vi "ContinousLoopMain.vi"(0 "ProgramPathInput":path, 11 "error in":errorcluster) -> (2 "Output Directory":path, 3 "File Prefix":string, 4 "Total Duration":dbl format="%<%H:%M:%S>t", 6 "Interval":dbl format="%<%H:%M:%S>t", 10 "Microscope":T1(array[cluster]), 12 "ProgramStopped":bool, 13 "StartProgram":bool, 14 "Positions":dbl[][](array[numeric]), 15 "error out":errorcluster)   [LabVIEW 2018, in "ContinousLoop.lvlib"]
uses:
  ContinousLoop.lvlib
  Config/Config.lvlib
panel:
  in  "Start Program":bool
  in  "stop":bool
  in  "Configuration File":path
  out "Continuous Program":string[][](array[string])
  # "Microscope"
  # "Program Control"
  # "Positions"
  # "Steps"
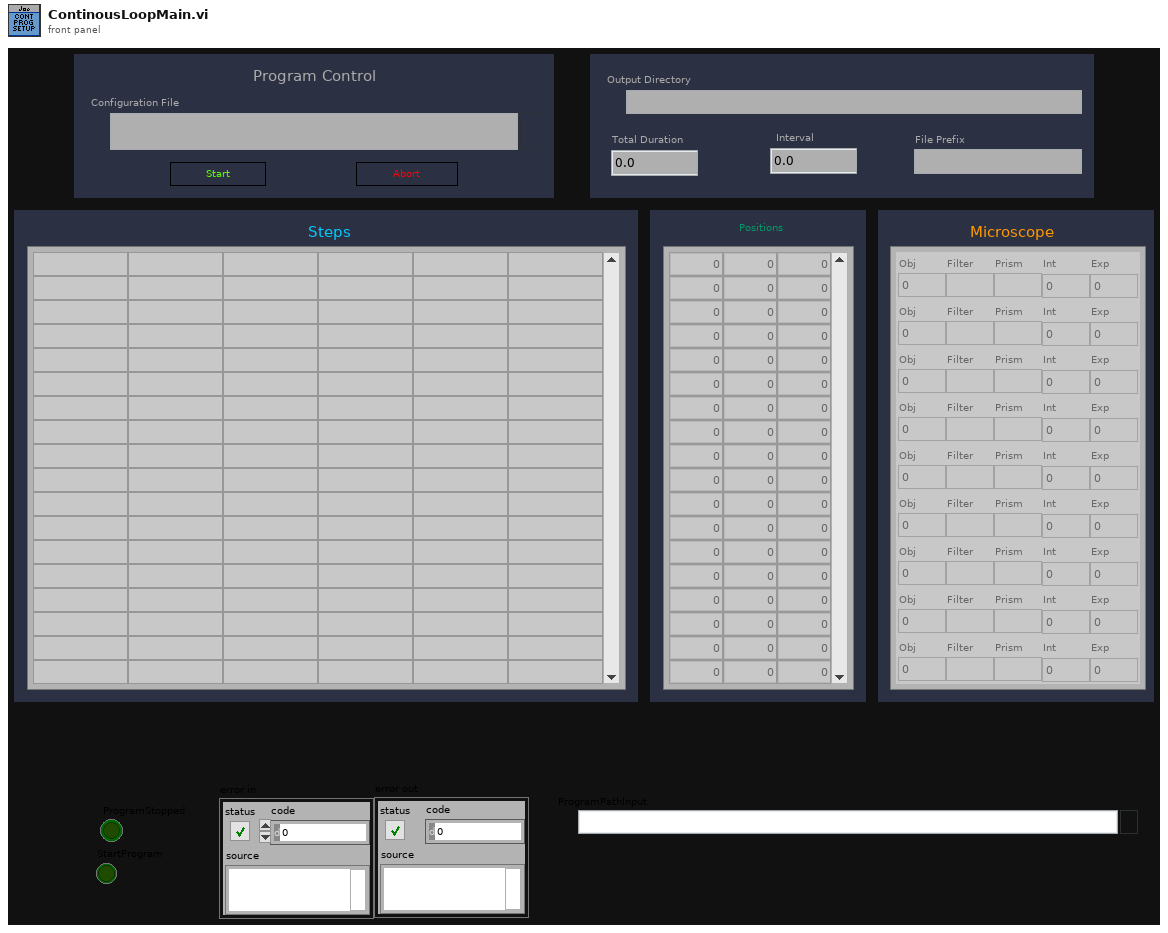
[diagram p1: front panel]
types:
  T1 = cluster{"Obj":i32, "Filter":string, "Prism":string, "Int":dbl, "Exp":i32}[]
  T2 = cluster{"Objective":i32, "Filter":string, "Prism":string, "Intensity":dbl, "Exposure":i32}[]
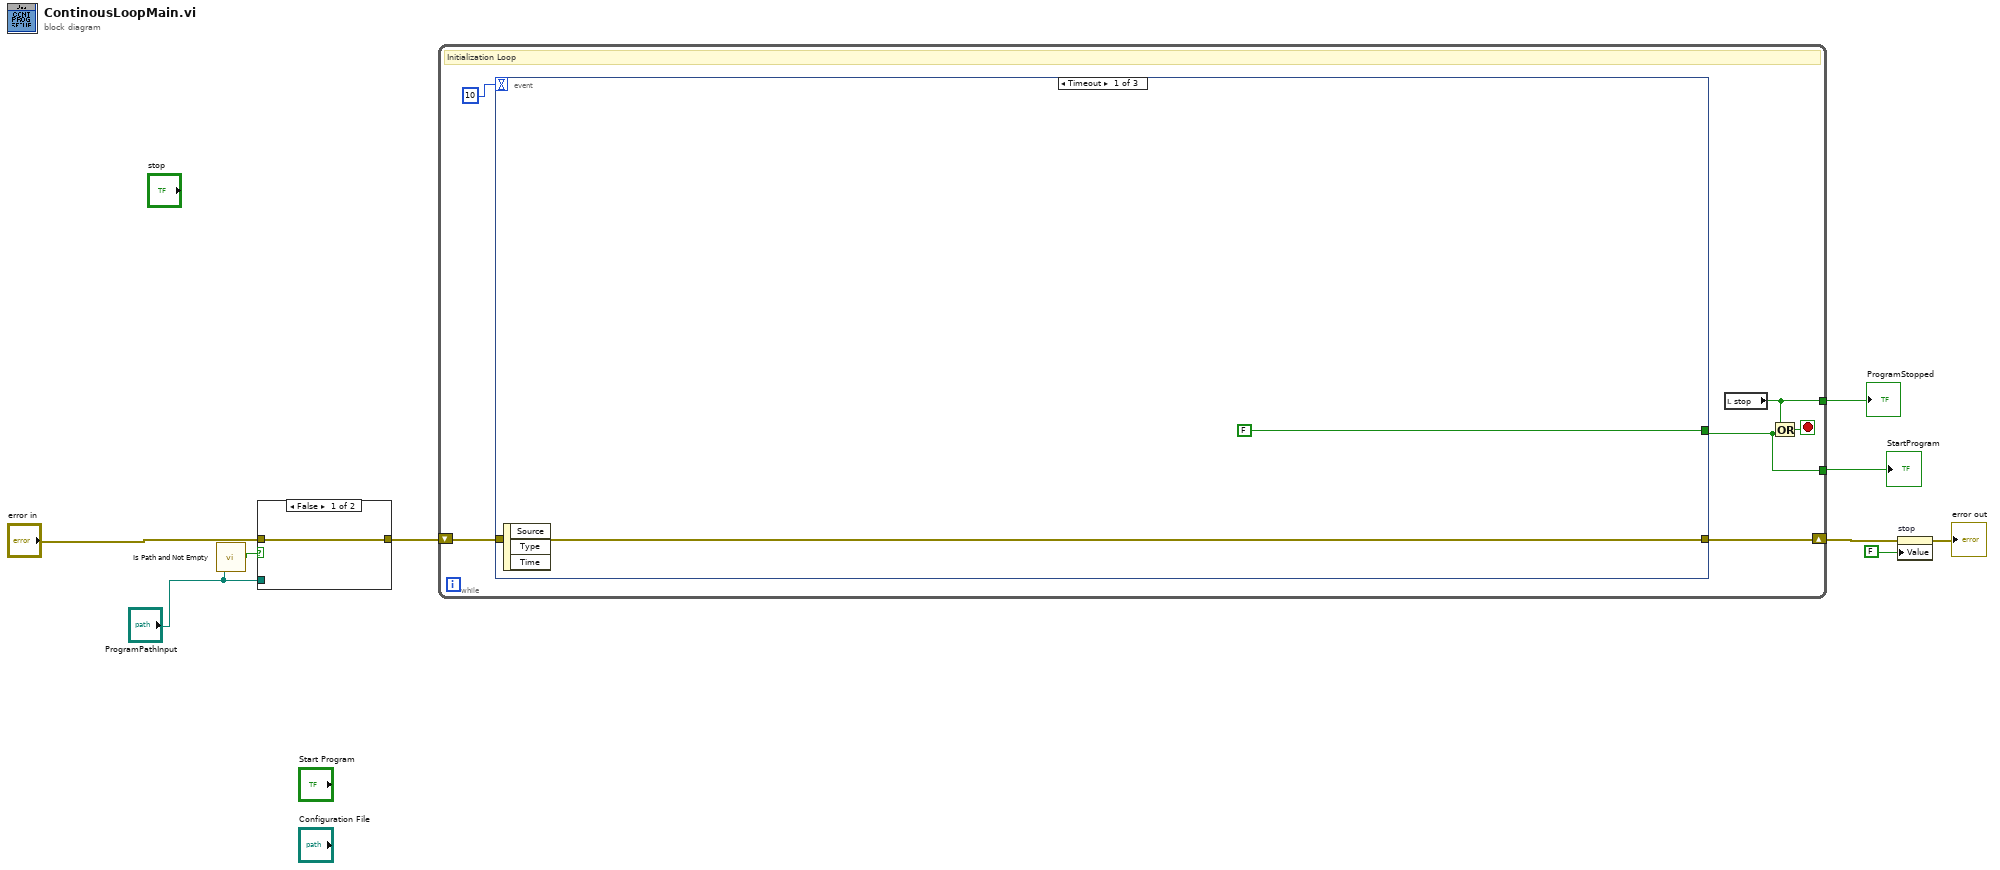
[diagram p0: block diagram]
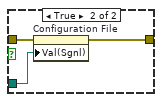
[diagram p2: hidden frame]
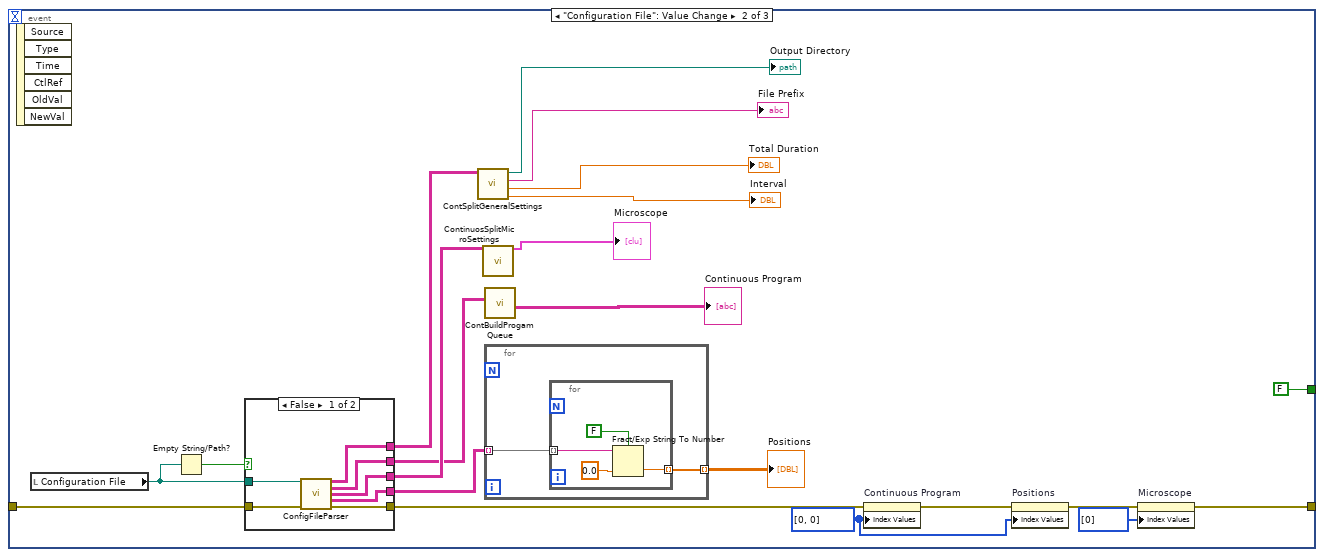
[diagram p3: hidden frame]
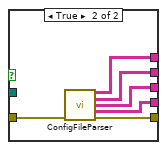
[diagram p4: hidden frame]
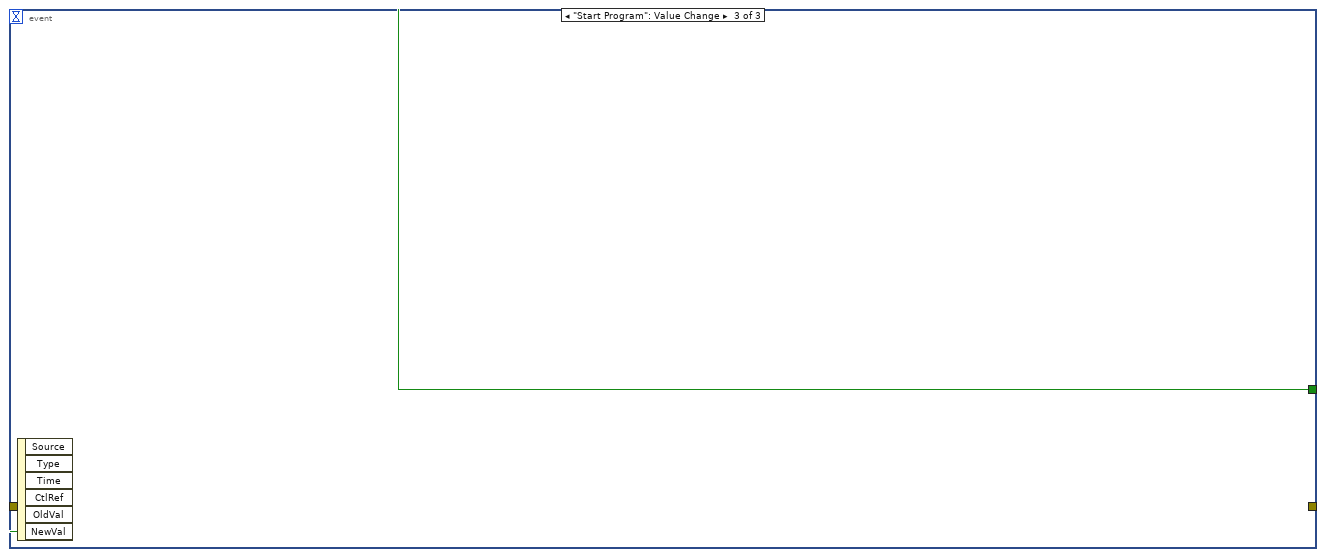
[diagram p5: hidden frame]
diagram:
  n1 = call <vilib>:"Is Path and Not Empty.vi"("path"="ProgramPathInput") -> ("Is Path and Not Empty?"=w5:bool)  [unwired: 4 in]
  n2 = case shown="False" w5 {
    tunnel: "error in" -> [w10 w13]
    tunnel: [w10 w12] -> w3
    tunnel: "ProgramPathInput" -> [_ w11]
    frame False {
    }
    frame True {
      n3 = property on="Configuration File" class="Path"(error in=w13, "Val(Sgnl)"=w11) -> (error out=w12:errorcluster)  [unwired: 1 in, 1 out]
    }
  }
  n4 = while {
    shift-right: [w18] -> w1
    shift-left: w3 -> [w17]
    tunnel: [w15] -> w7
    tunnel: [w14] -> w6
    stop <- w16 stop-if-true
    # "Initialization Loop"
    n5 = event shown="[0] Timeout" {
      selector: _ -> [_ _ _]
      dyn-events: _ -> [_ _ _]
      timeout: 10 -> [_ _ _]
      tunnel: [w21 w23 _] -> w18
      tunnel: w17 -> [w21 w34 _]
      tunnel: [FALSE ("NewVal") FALSE ("NewVal") w62] -> w15
      event Timeout {
        n6 = event-data() -> ()  [unwired: 1 in, 3 out]
      }
      event "Configuration File": Value Change {
        w24 = u32[] [0, 0] ("Index Values")
        n7 = event-data() -> ()  [unwired: 1 in, 6 out]
        n8 = local read "Configuration File"() -> (w39:path)
        n9 = Empty String/Path?(string/path=w39) -> (empty?=w40:bool)
        n10 = case shown="False" w40 {
          tunnel: w39 -> [w55 _]
          tunnel: [w54 w61] -> w35
          tunnel: [w53 w59] -> w41
          tunnel: [w52 w60] -> w38
          tunnel: [w51 w58] -> w37
          tunnel: [w50 w57] -> w28
          tunnel: w34 -> [w49 w56]
          frame False {
            n11 = call "ConfigFileParser.vi"("Path"=w55, "error in"=w49) -> ("General Settings"=w51:string[][], "Program"=w54:string[][], "Loop Microscope Settings"=w52:string[][], "Positions"=w53:string[][], "error out"=w50:errorcluster)  [unwired: 8 in, 1 out]
          }
          frame True {
            n12 = call "ConfigFileParser.vi"("error in"=w56) -> ("General Settings"=w58:string[][], "Program"=w61:string[][], "Loop Microscope Settings"=w60:string[][], "Positions"=w59:string[][], "error out"=w57:errorcluster)  [unwired: 9 in, 1 out]
          }
        }
        n13 = call "ContSplitGeneralSettings.vi"("General Settings"=w37) -> ("Interval"=→"Interval":dbl, "Total Duration"=→"Total Duration":dbl, "File Prefix"=→"File Prefix":string, "SaveDir"=→"Output Directory":path)  [unwired: 7 in]
        n14 = call "ContinuosSplitMicroSettings.vi"("Loop Microscope Settings"=w38) -> ("Microscope"=→"Microscope":T2)  [unwired: 14 in]
        n15 = call "ContBuildProgamQueue.vi"("Continuous Program"=w35) -> ("Continuous Program modified"=→"Continuous Program":string[][])  [unwired: 10 in]
        n16 = for {
          tunnel: w41 -> [w44] mode=indexing
          tunnel: [w43] -> w42 mode=indexing
          n17 = for {
            tunnel: w44 -> [w48] mode=indexing
            tunnel: [w47] -> w43 mode=indexing
            n18 = Fract/Exp String To Number(use system decimal point (T)=FALSE, string=w48, default (0 dbl)=0.0 ("default (0 DBL)")) -> (number=w47:dbl)  [unwired: 1 in, 1 out]
          }
        }
        "Positions" <- w42
        n19 = property on="Continuous Program" class="Arr (strict)"(error in=w28, "Index Values"=w24) -> (error out=w26:errorcluster)  [unwired: 1 in, 1 out]
        n20 = property on="Positions" class="Arr (strict)"(error in=w26, "Index Values"=w24) -> (error out=w25:errorcluster)  [unwired: 1 in, 1 out]
        n21 = property on="Microscope" class="Arr (strict)"(error in=w25, "Index Values"=u32[] [0]) -> (error out=w23:errorcluster)  [unwired: 1 in, 1 out]
      }
      event "Start Program": Value Change {
        n22 = event-data() -> ("NewVal"=w62:bool)  [unwired: 1 in, 5 out]
      }
    }
    n23 = local read "stop"() -> (w14:bool)
    n24 = Or(x=w14, y=w15) -> (x .or. y?=w16:bool)
  }
  "StartProgram" <- w7
  "ProgramStopped" <- w6
  n25 = property on="stop" class="Bool (strict)"(error in=w1, "Value"=FALSE ("stop")) -> (error out=→"error out":errorcluster)  [unwired: 1 in, 1 out]
